vi "IPS Ctrl Set Activity.vi"(3 "Error In":errorcluster={"status"=FALSE, "code"=1073676294, "source"="VISA Read in Prologix USB GPIB Command.vi"}, 4 "Activity":i32(listbox)=3, 5 "VISA resource name (COM Port of Prologix Device)":refnum<visa-resource-name>="GPIB1::25::INSTR") -> (0 "Error Out":errorcluster={"status"=TRUE, "code"=-1073807339, "source"="VISA Read in NI USB GPIB Command.vi->IPS Ctrl Set Activity.vi"}, 1 "Output":string="A\r", 2 "VISA resource name (COM Port of Prologix Device) 2":refnum<visa-resource-name>="GPIB1::25::INSTR")   [LabVIEW 2013]
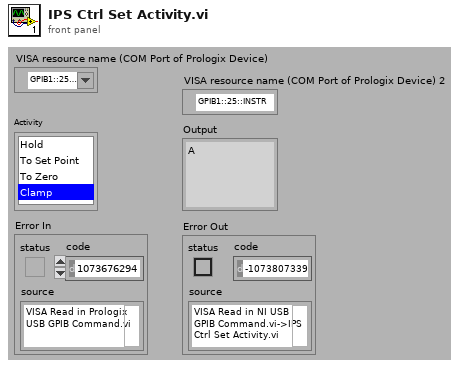
[diagram p1: front panel]
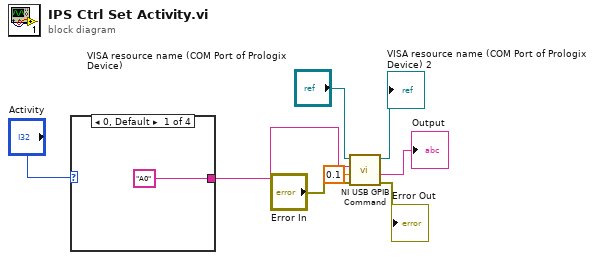
[diagram p0: block diagram]
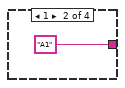
[diagram p2: hidden frame]
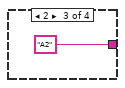
[diagram p3: hidden frame]
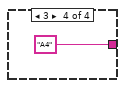
[diagram p4: hidden frame]
diagram:
  n1 = case shown="0, Default" "Activity" {
    tunnel: ["A0" "A1" "A2" "A4"] -> w3
    frame 0, Default {
    }
    frame 1 {
    }
    frame 2 {
    }
    frame 3 {
    }
  }
  n2 = call "NI USB GPIB Command.vi"("Error In"="Error In", "Wait for instrument to respond (s)"=0.1, "String to Send"=w3, "VISA resource name (COM Port of Prologix Device)"="VISA resource name (COM Port of Prologix Device)") -> ("Error Out"=→"Error Out":errorcluster, "Return String from Device (Not all commands return a String)"=→"Output":string, "VISA resource name (COM Port of Prologix Device) 2"=→"VISA resource name (COM Port of Prologix Device) 2":refnum<visa-resource-name>)  [unwired: 1 out]
